vi "Initialize Logger.vi"(8 "error in":errorcluster, 11 "Log Producer in":T1) -> (0 "error out":errorcluster, 3 "Log Producer out":T1)   [LabVIEW 2020, in "Frame Logging.lvlib"]
uses:
  Frame Logging.lvlib
  Log_Producer.ctl
  Message_Request.ctl
  Message_Request_Action.ctl
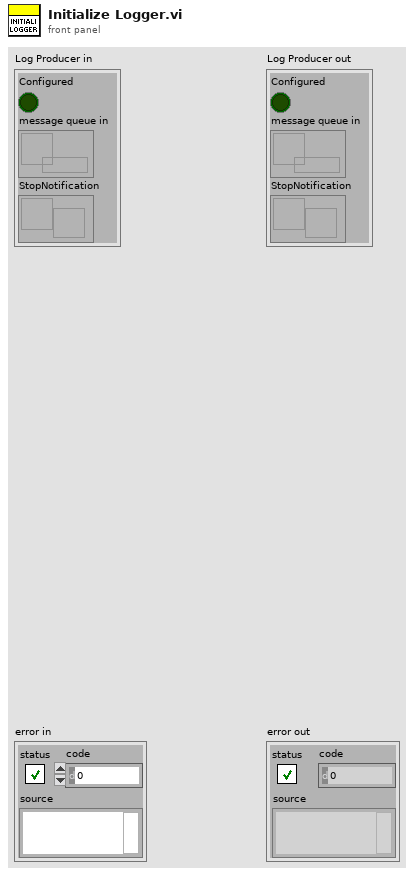
[diagram p1: front panel]
types:
  T1 = typedef "Frame Logging.lvlib/Log_Producer.ctl" = cluster{"Configured":bool, "message queue in":refnum<queue>, "StopNotification":refnum<notifier>}
  T2 = typedef "Frame Logging.lvlib/Message_Request_Action.ctl" = enum16{"Initialize", "Open File", "Log", "Manage Disk", "Stop", "Close File", "Update Configuration"}
  T3 = typedef "Frame Logging.lvlib/Message_Request.ctl" = cluster{"request":T2, "data":variant}
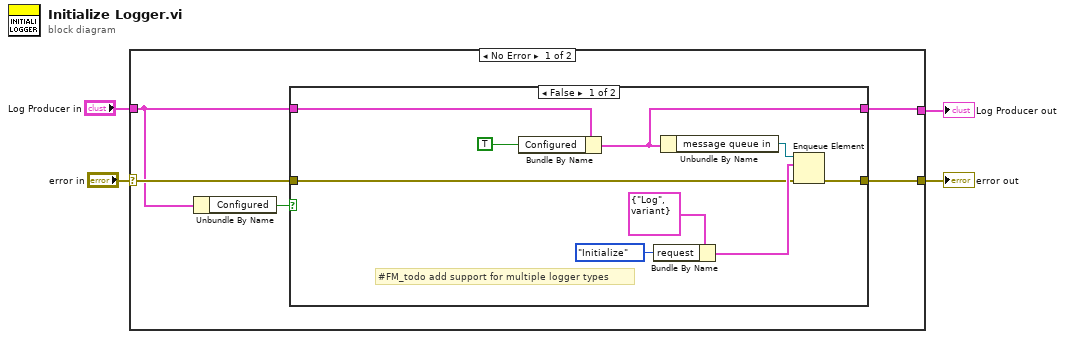
[diagram p0: block diagram]
diagram:
  n1 = case shown="No Error" "error in" {
    selector: "error in" -> [w9 w22]
    tunnel: [w8 w22] -> w3
    tunnel: [w6 w21] -> w1
    tunnel: "Log Producer in" -> [w7 w21]
    frame No Error {
      n2 = Unbundle By Name(w7) -> ("Configured"=w5:bool)
      n3 = case shown="False" w5 {
        tunnel: w9 -> [w10 w20]
        tunnel: [w16 w20] -> w8
        tunnel: w7 -> [w18 w19]
        tunnel: [w15 w19] -> w6
        frame False {
          # "#FM_todo add support for multiple logger types"
          n4 = Bundle By Name(cluster=w18, "Configured"=TRUE) -> (w15:T1)
          n5 = Bundle By Name(cluster=T3 {"request"=enum."Log", "data"=variant} ("element"), "request"=Message_Request_Action."Initialize") -> (w12:T3)
          n6 = Unbundle By Name(w15) -> ("message queue in"=w14:refnum<queue>)
          n7 = Enqueue Element(queue=w14, element=w12, error in (no error)=w10) -> (error out=w16:errorcluster)  [unwired: 1 in, 2 out]
        }
        frame True {
        }
      }
    }
    frame Error {
    }
  }
  "error out" <- w3
  "Log Producer out" <- w1
